vi "数据写入database.vi"(9 "data":variant, 10 "columns":string[](array[string]), 11 "table":string) -> (1 "error out":errorcluster)   [LabVIEW 2016, in "斯坦道CODMn.lvlib"]
uses:
  <vilib>/addons/database/Connection.llb/DB Tools Open Connec (String).vi
  <vilib>/addons/database/NI_Database_API.lvlib
panel:
  in  "error in (no error)":errorcluster
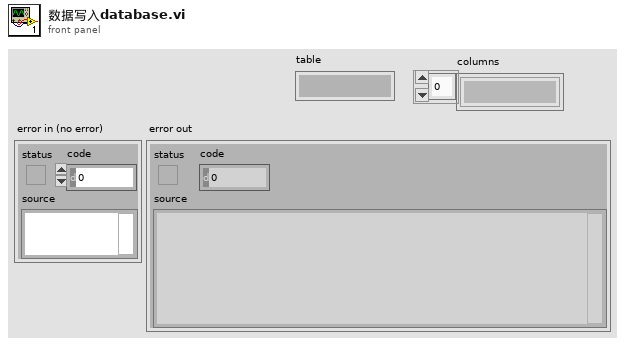
[diagram p1: front panel]
types:
  T1 = typedef "NI_Database_API.lvlib/Conn ObjectReference.ctl" = refnum<k1>
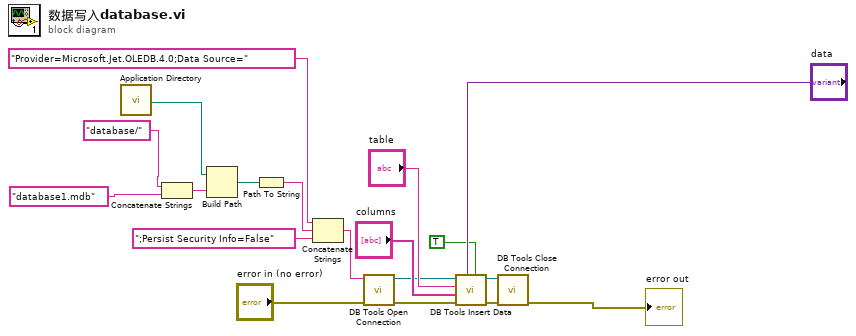
[diagram p0: block diagram]
diagram:
  n1 = call <vilib>:"Application Directory.vi"() -> ("Application Directory"=w1:path)
  n2 = Concatenate Strings("database/" ("condition"), "database1.mdb" ("字符串")) -> (w4:string)
  n3 = Build Path(base path=w1, name or relative path=w4) -> (appended path=w11:path)
  n4 = Path To String(path=w11) -> (string=w10:string)
  n5 = Concatenate Strings("Provider=Microsoft.Jet.OLEDB.4.0;Data Source=" ("condition"), w10, ";Persist Security Info=False" ("condition")) -> (w8:string)
  n6 = call-poly <vilib>:"DB Tools Open Connection.vi"("error in (no error)"="error in (no error)", "connection information"=w8) -> ("error out"=w5:errorcluster, "connection reference"=w6:T1)  [unwired: 6 in]
  n7 = call <vilib>:"DB Tools Insert Data.vi"("create table? (F)"=TRUE, "data"="data", "error in (no error)"=w5, "columns"="columns", "table"="table", "connection reference"=w6) -> ("error out"=w18:errorcluster, "connection reference out"=w19:T1)  [unwired: 4 in]
  n8 = call <vilib>:"DB Tools Close Connection.vi"("error in (no error)"=w18, "connection reference"=w19) -> ("error out"=→"error out":errorcluster)  [unwired: 5 in]
